vi "Sandbox.vi"() -> ()   [LabVIEW 2014]
uses:
  Controls/Attribute.ctl
  <vilib>/xml/Load XML File.vi
  <resource>/objmgr/DOMUserDefRef.rc
  <vilib>/xml/NI_XML.lvlib
  Controls/Node Type.ctl
panel:
  out "Local Name":string[][](array[string])
  out "Value":string[][](array[string])
  out "Type":i32[][](array[numeric])
  out "Name":string[][](array[string])
  in  "Attribute":T1
  out "Array 8":string[](array[string])
  out "Array 7":string[](array[string])
  out "Array 6":i32[](array[numeric])
  out "Array 5":string[](array[string])
  in  "path to XML document 2":path=path "C:/Users/rmowb/Desktop/NGI Sound Test 2.4.6.7.xml" caption="path to XML document"
  in  "Node":refnum<k20>
  in  "path to XML document":path=path "C:/Users/rmowb/Documents/_Code/XML Editor/Editor.xml"
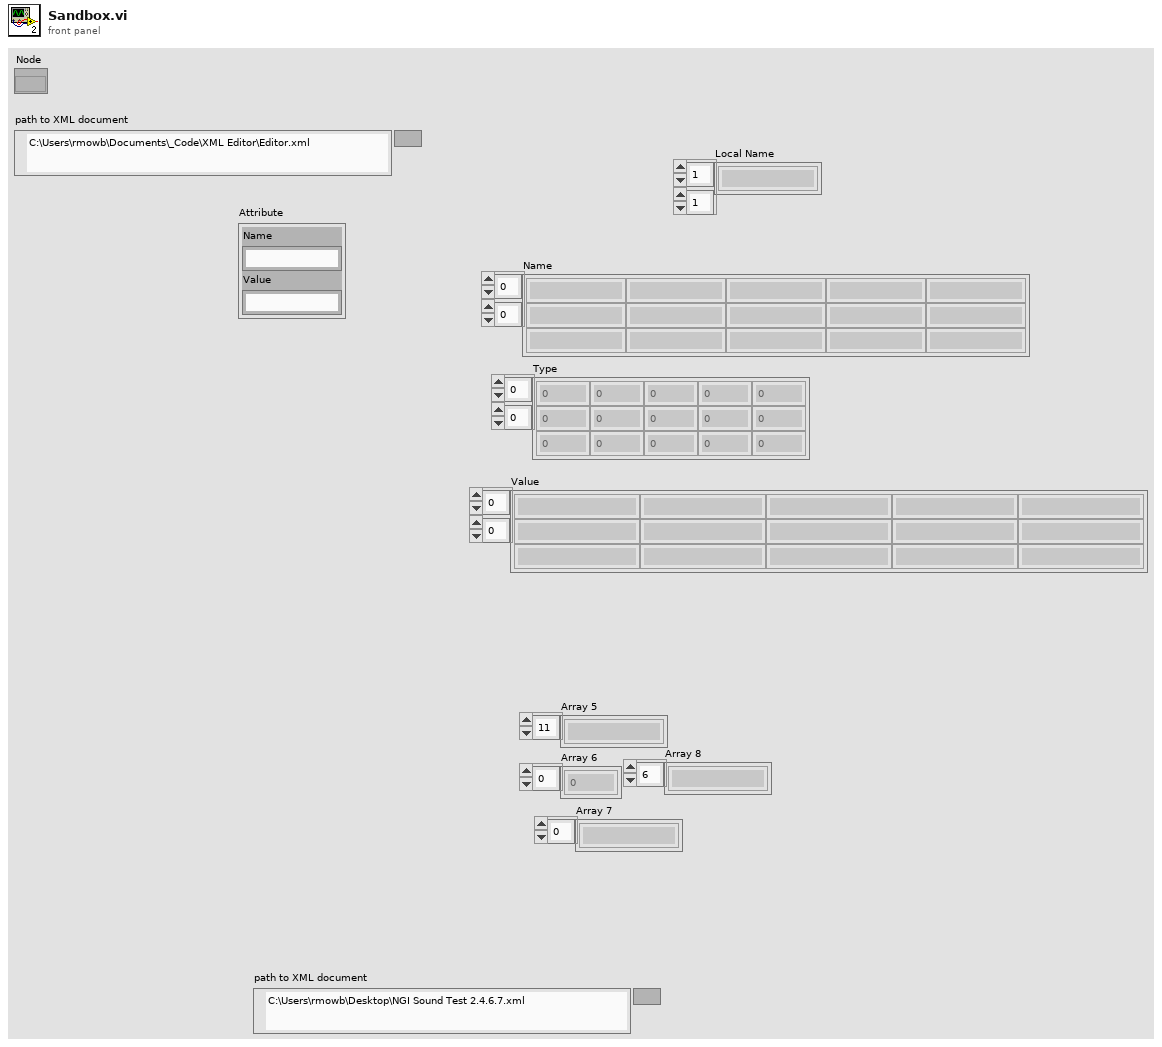
[diagram p1: front panel]
types:
  T1 = typedef "Attribute.ctl" = cluster{"Name":string, "Value":string}
  T2 = typedef "Node Type.ctl" = i32
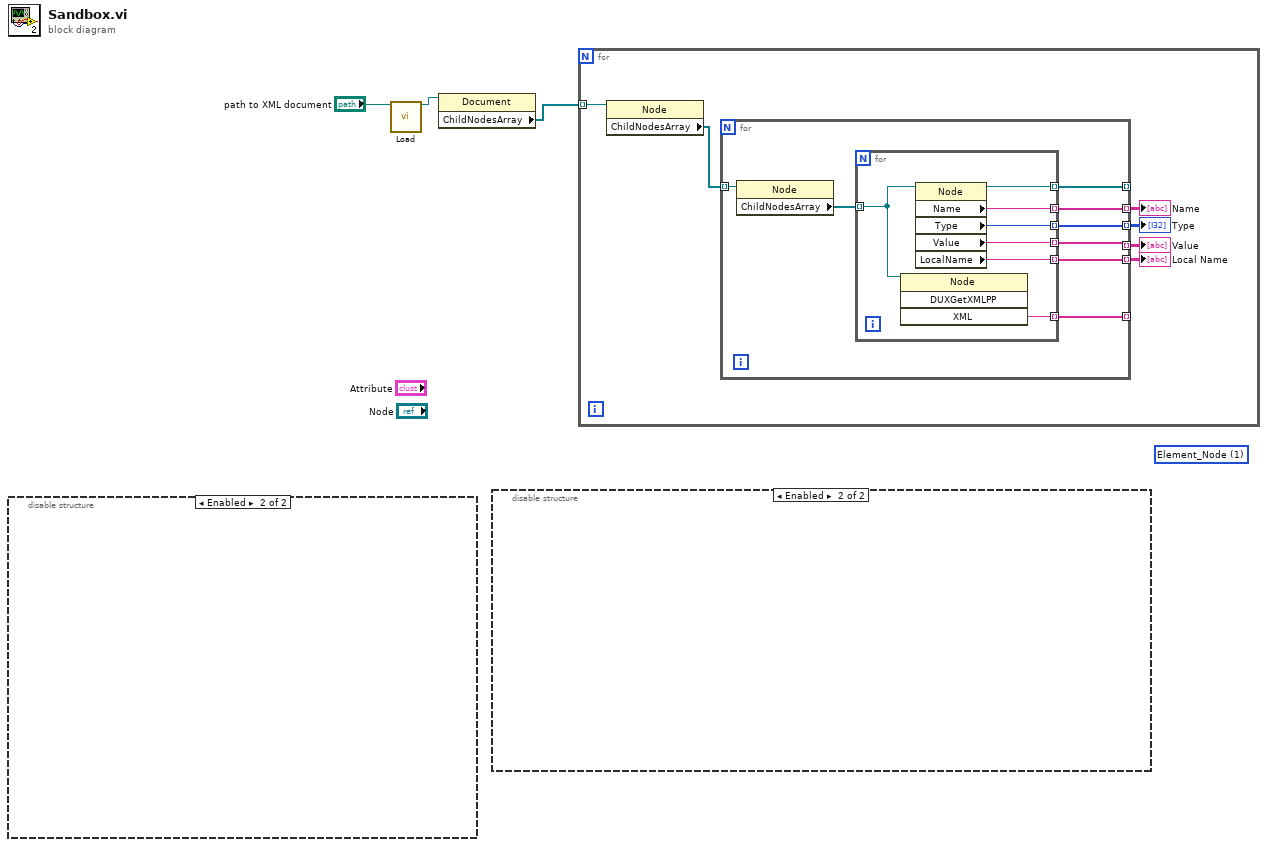
[diagram p0: block diagram]
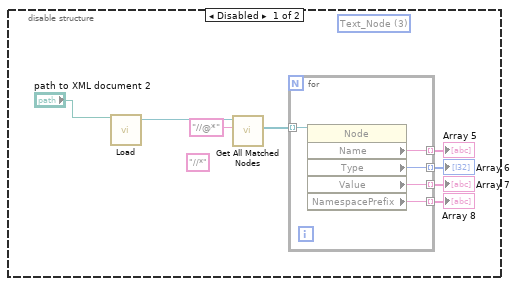
[diagram p2: hidden frame]
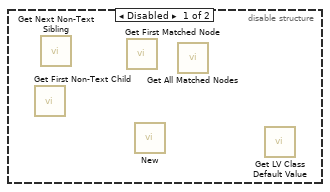
[diagram p3: hidden frame]
diagram:
  (unwired) 1 items=["Element_Node"=1, "Attribute_Node"=2, "Text_Node"=3, "CDATASection_Node"=4, "EntityReference_Node"=5, "Entity_Node"=6, "ProcessingInstruction_Node"=7, "Comment_Node"=8, "Document_Node"=9, "DocumentType_Node"=10, "DocumentFragment_Node"=11, "Notation_Node"=12] ("Node Type")
  n1 = disable-structure shown="Enabled" {
    frame Disabled {
      n2 = call <vilib>:"Get First Non-Text Child.vi"() -> ()  [unwired: 8 in, 4 out]
      n3 = call <vilib>:"Get Next Non-Text Sibling.vi"() -> ()  [unwired: 8 in, 4 out]
      n4 = call <vilib>:"Get First Matched Node.vi"() -> ()  [unwired: 9 in, 3 out]
      n5 = call <vilib>:"New.vi"() -> ()  [unwired: 8 in, 2 out]
      n6 = call <vilib>:"Get All Matched Nodes.vi"() -> ()  [unwired: 9 in, 3 out]
      n7 = call <vilib>:"Get LV Class Default Value.vi"() -> ()  [unwired: 10 in, 2 out]
    }
    frame Enabled {
    }
  }
  n8 = call-poly <vilib>:"Load.vi"("path to XML document"="path to XML document") -> ("DOM document out"=w1:refnum<k20>)  [unwired: 12 in, 2 out]
  n9 = property class="Document"(reference=w1) -> ("ChildNodesArray"=w2:refnum<k20>[])  [unwired: 1 in, 2 out]
  n10 = disable-structure shown="Enabled" {
    frame Disabled {
      (unwired) "//*" ("XPath expression")
      (unwired) T2 3 items=["Element_Node"=1, "Attribute_Node"=2, "Text_Node"=3, "CDATASection_Node"=4, "EntityReference_Node"=5, "Entity_Node"=6, "ProcessingInstruction_Node"=7, "Comment_Node"=8, "Document_Node"=9, "DocumentType_Node"=10, "DocumentFragment_Node"=11, "Notation_Node"=12] ("Node Type")
      n11 = call-poly <vilib>:"Load.vi"("path to XML document"="path to XML document 2") -> ("DOM document out"=w10:refnum<k20>)  [unwired: 12 in, 2 out]
      n12 = call <vilib>:"Get All Matched Nodes.vi"("XPath expression"="//@*", "node in"=w10) -> ("node result array"=w8:refnum<k20>[])  [unwired: 7 in, 2 out]
      n13 = for {
        tunnel: w8 -> [w16] mode=indexing
        tunnel: [w15] -> w7 mode=indexing
        tunnel: [w14] -> w6 mode=indexing
        tunnel: [w13] -> w5 mode=indexing
        tunnel: [w12] -> w4 mode=indexing
        n14 = property class="Node"(reference=w16) -> ("Name"=w15:string, "Type"=w14:i32, "Value"=w13:string, "NamespacePrefix"=w12:string)  [unwired: 1 in, 2 out]
      }
      "Array 5" <- w7
      "Array 6" <- w6
      "Array 7" <- w5
      "Array 8" <- w4
    }
    frame Enabled {
    }
  }
  n15 = for {
    tunnel: w2 -> [w17] mode=indexing
    n16 = property class="Node"(reference=w17) -> ("ChildNodesArray"=w22:refnum<k20>[])  [unwired: 1 in, 2 out]
    n17 = for {
      tunnel: w22 -> [w25] mode=indexing
      tunnel: [w30] -> w21 mode=indexing
      tunnel: [w29] -> _ mode=indexing
      tunnel: [w28] -> w20 mode=indexing
      tunnel: [w27] -> w19 mode=indexing
      tunnel: [w26] -> _ mode=indexing
      tunnel: [w23] -> w18 mode=indexing
      n18 = property class="Node"(reference=w25) -> ("ChildNodesArray"=w24:refnum<k20>[])  [unwired: 1 in, 2 out]
      n19 = for {
        tunnel: [w37] -> w30 mode=indexing
        tunnel: [w36] -> w29 mode=indexing
        tunnel: [w35] -> w28 mode=indexing
        tunnel: [w34] -> w27 mode=indexing
        tunnel: [w33] -> w26 mode=indexing
        tunnel: w24 -> [w32] mode=indexing
        tunnel: [w31] -> w23 mode=indexing
        n20 = invoke class="Node" method="DUXGetXMLPP"(reference=w32) -> ("XML"=w33:string)  [unwired: 3 in, 3 out]
        n21 = property class="Node"(reference=w32) -> (reference out=w36:refnum<k20>, "Name"=w37:string, "Type"=w35:i32, "Value"=w34:string, "LocalName"=w31:string)  [unwired: 1 in, 1 out]
      }
    }
    "Name" <- w21
    "Type" <- w20
    "Value" <- w19
    "Local Name" <- w18
  }
